vi "Pockels Cal-Wizard window.vi"(8 "error in (no error)":errorcluster) -> (0 "error out":errorcluster, 1 "Cancelled":bool)   [LabVIEW 2020]
doc: "Use this template to create a dialog box with event handling."
uses:
  AOL Z/Typedefs/Cal mode.ctl
  AOL Z/Typedefs/Pre-AOL Z wizard refs.ctl
  <vilib>/Utility/miscctls.llb/LVPointTypeDef.ctl
  Typedefs/Colapsed-Expanded.ctl
  Global Variables/General Globals.vi
  Globals/gl_Calibration globals.vi
panel:
  out "2D Picture":picture
  in  "Power meter AI":tag
  out "Message":string
  in  "Calibration Mode":T1
  in  "Back":bool
  in  "Next":bool
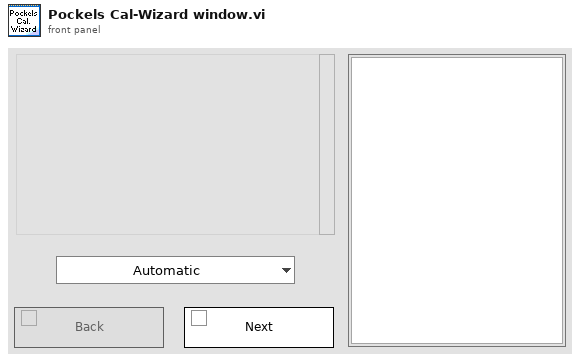
[diagram p1: front panel]
types:
  T1 = typedef "Cal mode.ctl" = enum16{"Automatic", "Interactive"}
  T2 = typedef "Pre-AOL Z wizard refs.ctl" = cluster{"VI's reference":refnum<vi>, "Calibration Mode":refnum<vi>, "Cal points":refnum<vi>, "Channel Selector":refnum<vi>, "Message":refnum<vi>, "Back":refnum<vi>, "Next":refnum<vi>, "Power meter AI":refnum<vi>, "2D Picture":refnum<vi>, "Note":refnum<vi>}
  T3 = typedef "Pockels cal wizard states.ctl" = enum16{"Select cal mode", "Show instructions 1", "Select channel", "Show instructions 2", "Show instructions 3", "Confirm start", "Start calibration"}
  T4 = typedef "LVPointTypeDef.ctl" = cluster{"Horizontal":i16, "Vertical":i16}
  T5 = typedef "LVRectTypeDef.ctl" = cluster{"Left":i16, "Top":i16, "Right":i16, "Bottom":i16}
  T6 = typedef "Colapsed-Expanded.ctl" = enum16{"Original size", "Expanded-Size A"}
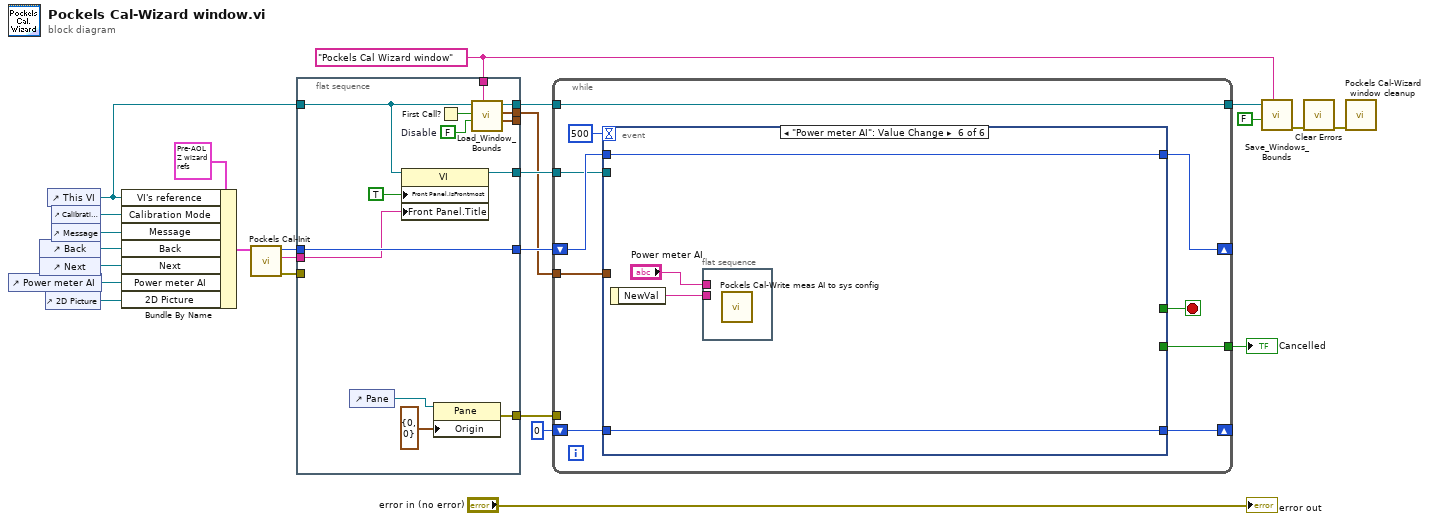
[diagram p0: block diagram]
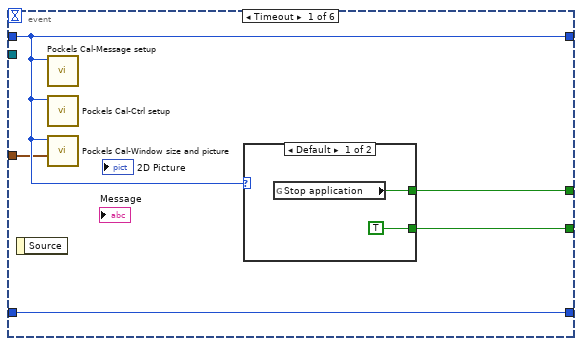
[diagram p2: hidden frame]
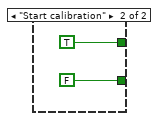
[diagram p3: hidden frame]
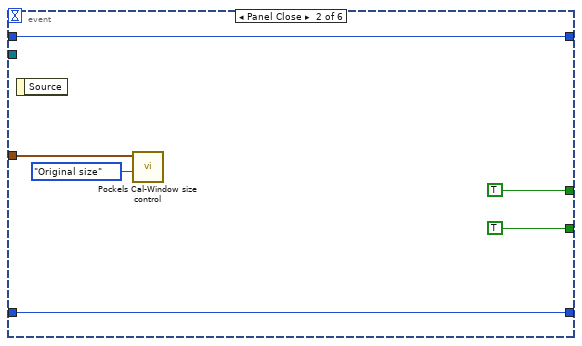
[diagram p4: hidden frame]
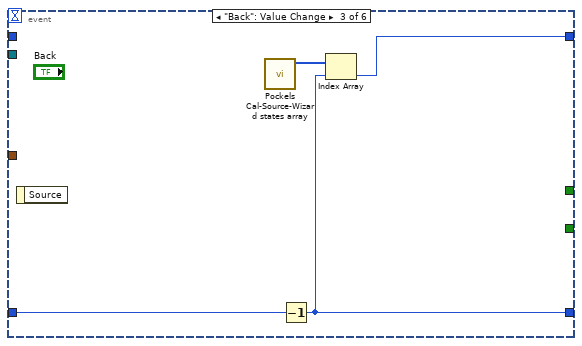
[diagram p5: hidden frame]
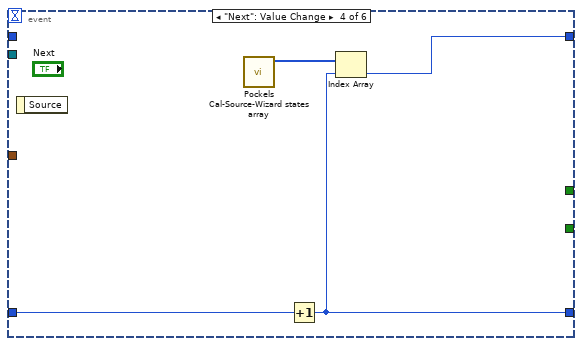
[diagram p6: hidden frame]
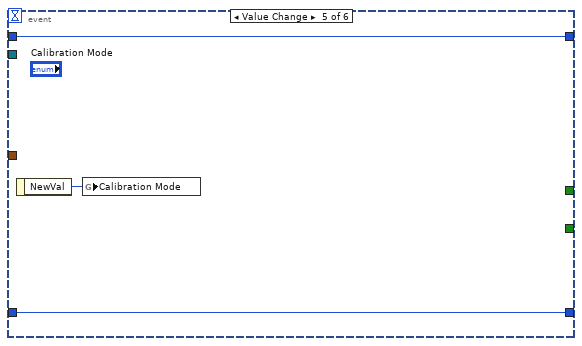
[diagram p7: hidden frame]
diagram:
  w15 = "Pockels Cal Wizard window" ("Window Name (i.e. Key)")
  n1 = control-ref of="Power meter AI"() -> (w7:refnum<vi>)
  n2 = control-ref of="Back"() -> (w12:refnum<vi>)
  n3 = control-ref of="Next"() -> (w11:refnum<vi>)
  n4 = control-ref of="2D Picture"() -> (w4:refnum<vi>)
  n5 = control-ref of="This VI"() -> (w3:refnum<vi>)
  n6 = control-ref of="Calibration Mode"() -> (w18:refnum<vi>)
  n7 = control-ref of="Message"() -> (w13:refnum<vi>)
  n8 = Bundle By Name(cluster=T2 {"VI's reference"=refnum, "Calibration Mode"=refnum, "Cal points"=refnum, "Channel Selector"=refnum, "Message"=refnum, "Back"=refnum, "Next"=refnum, "Power meter AI"=refnum, "2D Picture"=refnum, "Note"=refnum} ("Pre-AOL Z wizard refs"), "VI's reference"=w3, "Calibration Mode"=w18, "Message"=w13, "Back"=w12, "Next"=w11, "Power meter AI"=w7, "2D Picture"=w4) -> (w16:T2)
  n9 = call "Pockels Cal-Init.vi"("Pre-AOL Z wizard refs"=w16) -> ("error out"=w14:errorcluster, "Cal settings window's title"=w9:string, "Initial state"=w10:T3)  [unwired: 8 in]
  n10 = flat-sequence {
    tunnel: [w38] -> w25
    tunnel: [w36] -> w24
    tunnel: [w32] -> w22
    tunnel: [w30] -> w8
    tunnel: w15 -> [w31]
    tunnel: w14 -> [_]
    tunnel: w10 -> [w30]
    tunnel: w9 -> [w29]
    tunnel: w3 -> [w26]
    tunnel: [w28] -> w5
    tunnel: [w27] -> _
    frame #0 {
      w33 = FALSE  # Disable
      n11 = control-ref of="Pane"() -> (w35:refnum<vi>)
      n12 = property on="Property Node" class="VI"(reference=w26, "Front Panel.IsFrontmost"=TRUE ("Front Panel Window:Is Frontmost"), "Front Panel.Title"=w29) -> (reference out=w38:refnum<vi>)  [unwired: 1 in, 1 out]
      n13 = property class="Pane"(reference=w35, "Origin"=T4 {"Horizontal"=0, "Vertical"=0}) -> (error out=w36:errorcluster)  [unwired: 1 in, 1 out]
      n14 = First Call?() -> (First Call?: T/F=w34:bool)
      n15 = call "Load_Window_Bounds.vi"("Window Name (i.e. Key)"=w31, "Disable"=w33, "First Call"=w34, "Window VI's Ref"=w26) -> ("Front Panel.WinBounds"=w27:T5, "Window size"=w28:cluster{"Horisontal":i16, "Vertical":i16}, "reference out"=w32:refnum<vi>)  [unwired: 4 in, 1 out]
    }
  }
  n16 = while {
    tunnel: w24 -> [_]
    tunnel: w25 -> [w40]
    tunnel: [w47] -> w19
    tunnel: w22 -> [w46]
    tunnel: [w46] -> w21
    shift-right: [w44] -> _
    shift-left: w8 -> [w45]
    shift-right: [w42] -> _
    shift-left: 0 -> [w43]
    tunnel: w5 -> [w41]
    stop <- w49 stop-if-true
    n17 = event shown="[5] \"Power meter AI\": Value Change" {
      selector: _ -> [_ _ _ _ _ _]
      dyn-events: _ -> [_ _ _ _ _ _]
      timeout: 500 -> [_ _ _ _ _ _]
      tunnel: [w54 TRUE ("Stop?") _ _ _ _] -> w49
      tunnel: [w53 TRUE ("Stop subpanel") _ _ _ _] -> w47
      tunnel: w45 -> [w51 w62 _ _ w75 w79]
      tunnel: [w51 w62 w67 w71 w75 w79] -> w44
      tunnel: w43 -> [w52 w61 w66 w70 w73 w78]
      tunnel: [w52 w61 w65 w69 w73 w78] -> w42
      tunnel: w41 -> [w50 w60 _ _ _ _]
      tunnel: w40 -> [_ _ _ _ _ _]
      event Timeout {
        n18 = event-data() -> ()  [unwired: 1 in, 1 out]
        n19 = call "Pockels Cal-Message setup.vi"("State"=w51) -> ()  [unwired: 10 in, 1 out]
        n20 = call "Pockels Cal-Ctrl setup.vi"("State"=w51) -> ()  [unwired: 10 in, 1 out]
        n21 = call "Pockels Cal-Window size and picture.vi"("Original window size"=w50, "State"=w51) -> ()  [unwired: 9 in, 1 out]
        n22 = case shown="Default" w51 {
          tunnel: [w56 TRUE] -> w54
          tunnel: [TRUE ("Stop application") FALSE ("Stop application")] -> w53
          frame Default {
            n23 = global read "General Globals.vi" "Stop application"() -> (w56:bool)
          }
          frame "Start calibration" {
          }
        }
      }
      event Panel Close {
        n24 = event-data() -> ()  [unwired: 1 in, 1 out]
        n25 = call "Pockels Cal-Window size control.vi"("Function"=Colapsed-Expanded."Original size", "Original window size"=w60) -> ()  [unwired: 9 in, 1 out]
      }
      event "Back": Value Change {
        n26 = event-data() -> ()  [unwired: 1 in, 1 out]
        n27 = call "Pockels Cal-Source-Wizard states array.vi"() -> ("States sequence"=w68:T3[])  [unwired: 11 in]
        n28 = Decrement(x=w66) -> (x-1=w65:i32)
        n29 = Index Array(array=w68, index=w65) -> (element=w67:T3)
      }
      event "Next": Value Change {
        n30 = event-data() -> ()  [unwired: 1 in, 1 out]
        n31 = call "Pockels Cal-Source-Wizard states array.vi"() -> ("States sequence"=w72:T3[])  [unwired: 11 in]
        n32 = Increment(x=w70) -> (x+1=w69:i32)
        n33 = Index Array(array=w72, index=w69) -> (element=w71:T3)
      }
      event Value Change {
        n34 = event-data() -> ("NewVal"=w74:T1)  [unwired: 1 in]
        n35 = global write "gl_Calibration globals.vi" "Calibration Mode"(w74) -> ()
      }
      event "Power meter AI": Value Change {
        n36 = event-data() -> ("NewVal"=w77:tag)  [unwired: 1 in]
        n37 = flat-sequence {
          tunnel: w77 -> [_]
          tunnel: "Power meter AI" -> [_]
          frame #0 {
            n38 = call "Pockels Cal-Write meas AI to sys config.vi"() -> ()  [unwired: 11 in, 1 out]
          }
        }
      }
    }
  }
  "Cancelled" <- w19
  n39 = call "Save_Windows_Bounds.vi"("Window Name (i.e. Key)"=w15, "Front Panel Window:Open"=FALSE, "Window VI's Ref"=w21) -> ("Error out (pass-through)"=w2:errorcluster)  [unwired: 8 in]
  n40 = call <vilib>:"Clear Errors.vi"("error in (no error)"=w2) -> ("error out"=w1:errorcluster)  [unwired: 5 in, 1 out]
  n41 = call "Pockels Cal-Wizard window cleanup.vi"("error in (no error)"=w1) -> ()  [unwired: 11 in]
  "error out" <- "error in (no error)"
